vi "InRangeImageARGB.vi"(8 "error in (no error)":errorcluster, 9 "In-Range Image Colour Range":T1, 10 "In-Range-Result":refnum<data-value>, 11 "ARGB Image Source":refnum<data-value>) -> (0 "error out":errorcluster, 3 "In-Range-Result (duplicate)":refnum<data-value>)   [LabVIEW 2020, in "g_ar_toolkit.image.lvlib"]
uses:
  g_ar_toolkit.image.lvlib
  In-Range Image Colour Range.ctl
  <vilib>/Utility/error.llb/Error Cluster From Error Code.vi
  ffccc43a-a069-4092-9152-56f2c6e40fec.vi
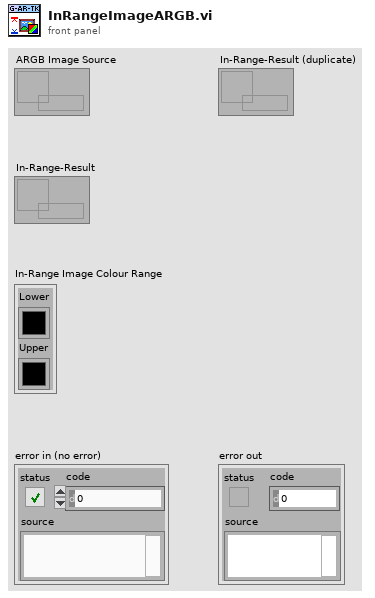
[diagram p1: front panel]
types:
  T1 = typedef "g_ar_toolkit.image.lvlib/In-Range Image Colour Range.ctl" = cluster{"Lower":u32, "Upper":u32}
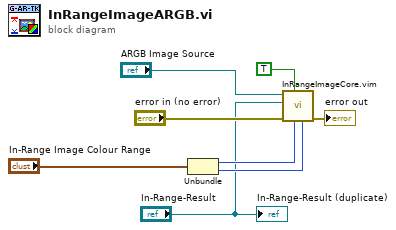
[diagram p0: block diagram]
diagram:
  n1 = Unbundle("In-Range Image Colour Range") -> ("Lower"=w6:u32, "Upper"=w5:u32)
  n2 = call "InRangeImageCore.vim"("Upper"=w5, "Lower"=w6, "IgnoreAlpha"=TRUE, "error in (no error)"="error in (no error)", "In-Range-Result"="In-Range-Result", "Src"="ARGB Image Source") -> ("error out"=→"error out":errorcluster)  [unwired: 5 in]
  "In-Range-Result (duplicate)" <- "In-Range-Result"
